vi "NI 9775 Continuous Mode 4 channels (Host).vi"() -> ()   [LabVIEW 2021]
uses:
  <vilib>/userDefined/High Color/nirio_resource_hc.ctl
  <vilib>/LabVIEW Targets/FPGA/cRIO/shared/nicrio_ModuleControls/nicrio_cRIO-9775_ContinuousDataRates4ChansRing.ctl
  <vilib>/LabVIEW Targets/FPGA/cRIO/shared/nicrio_ModuleControls/nicrio_BasicConversionTime.ctl
  <vilib>/FPGAPlugInAG/cRIO-9053/niLvFpga_Open_cRIO-9053.vi
  <vilib>/rvi/interface/common/dynamic/niFpgaDynamicAddResources.vi
  <vilib>/FPGAPlugInAG/Dynamic/niLvFpga_Reset_Dynamic.vi
  <vilib>/Utility/error.llb/Error Cluster From Error Code.vi
  <vilib>/rvi/errors/niLvFpgaAdjustHostInterfaceError.vi
  <vilib>/FPGAPlugInAG/Dynamic/niLvFpga_Run_Dynamic.vi
  <vilib>/Utility/file.llb/Write Delimited Spreadsheet (DBL).vi
  <vilib>/FPGAPlugInAG/Dynamic/niLvFpga_Close_Dynamic.vi
  <vilib>/rvi/interface/nirviOpenFPGA/nirviOpenFPGA.xnode
  FPGA Bitfiles/ni9775crio9053_FPGATarget2_NI9775GettingSta_I+1qGd-Sz4M.lvbitx
  <vilib>/rvi/interface/nirviMethod/nirviMethod.xnode
  <vilib>/rvi/interface/nirviReadWriteControl/nirviReadWriteControl.xnode
  <vilib>/rvi/interface/nirviCloseFPGA/nirviCloseFPGA.xnode
  <vilib>/rvi/interface/Simulation/niFpgaSimulationCallBeginRW.vi
  <vilib>/FPGAPlugInAG/Dynamic/niLvFpga_ReadFifo_Dynamic.vi
  <vilib>/rvi/errors/niLvFpgaMergeErrorWithErrorCode.vi
  NiFpgaLv.dll
panel:
  out "Num pts Pos":i32=50
  out "Modulation frequency":dbl=1000.0
  out "Sample Rate":dbl=100000.0
  out "Num pts Neg":i32=50
  out "Raw signal":waveform(dbl)[](graph)=[{"t0"=timestamp(0 s since 1904-01-01), "dt"=1e-05, "Y"=array[4941 elements]}, {"t0"=timestamp(0 s since 1904-01-01), "dt"=1e-05, "Y"=array[4941 elements]}, {"t0"=timestamp(0 s since 1904-01-01), "dt"=1e-05, "Y"=array[4941 elements]}, {"t0"=timestamp(0 s since 1904-01-01), "dt"=1e-05, "Y"=array[4941 elements]}]
  in  "Save modulated signal":bool=TRUE
  out "Producer loop time":u32=50
  out "Consumer loop time":u32=50
  in  "Filename":path=path "C:/Users/data/ni9775_100ks_1khz.lvm"
  in  "Consumer loop update rate (ms)":u32=10
  out "Demodulated Signal":dbl(graph)
  out "middle point pos":dbl=0.437255859375
  out "Queue":i32
  out "Original Signal middle":dbl(graph)=0.437255859375
  out "Low level":bool=TRUE
  out "High level":bool
  in  "Enable Low Pass Filter":T1={"Enable Low Pass Filter CH1"=TRUE, "Enable Low Pass Filter CH2"=TRUE, "Enable Low Pass Filter CH3"=TRUE, "Enable Low Pass Filter CH0"=TRUE}
  in  "Timing Mode":T2=enum."High Resolution"
  in  "Continuous Data Rate":T3=200 items=["1.000 MS/s (NI 9775)"=20, "833.333 KS/s (NI 9775)"=24, "714.286 KS/s (NI 9775)"=28, "625.000 KS/s (NI 9775)"=32, "555.556 KS/s (NI 9775)"=36, "500.000 KS/s (NI 9775)"=40, "454.545 KS/s (NI 9775)"=44, "416.667 KS/s (NI 9775)"=48, "384.615 KS/s (NI 9775)"=52, "357.143 KS/s (NI 9775)"=56, "333.333 KS/s (NI 9775)"=60, "312.500 KS/s (NI 9775)"=64, "294.118 KS/s (NI 9775)"=68, "277.778 KS/s (NI 9775)"=72, "263.158 KS/s (NI 9775)"=76, "250.000 KS/s (NI 9775)"=80, "238.095 KS/s (NI 9775)"=84, "227.273 KS/s (NI 9775)"=88, "217.391 KS/s (NI 9775)"=92, "208.333 KS/s (NI 9775)"=96, "200.000 KS/s (NI 9775)"=100, "192.308 KS/s (NI 9775)"=104, "185.185 KS/s (NI 9775)"=108, "178.571 KS/s (NI 9775)"=112, "172.414 KS/s (NI 9775)"=116, "166.667 KS/s (NI 9775)"=120, "161.290 KS/s (NI 9775)"=124, "156.250 KS/s (NI 9775)"=128, "151.515 KS/s (NI 9775)"=132, "147.059 KS/s (NI 9775)"=136, "142.857 KS/s (NI 9775)"=140, "138.889 KS/s (NI 9775)"=144, "135.135 KS/s (NI 9775)"=148, "131.579 KS/s (NI 9775)"=152, "128.205 KS/s (NI 9775)"=156, "125.000 KS/s (NI 9775)"=160, "121.951 KS/s (NI 9775)"=164, "119.048 KS/s (NI 9775)"=168, "116.279 KS/s (NI 9775)"=172, "113.636 KS/s (NI 9775)"=176, "111.111 KS/s (NI 9775)"=180, "108.696 KS/s (NI 9775)"=184, "106.383 KS/s (NI 9775)"=188, "104.167 KS/s (NI 9775)"=192, "102.041 KS/s (NI 9775)"=196, "100.000 KS/s (NI 9775)"=200, "50.000 KS/s (NI 9775)"=400, "33.333 KS/s (NI 9775)"=600, "25.000 KS/s (NI 9775)"=800, "20.000 KS/s (NI 9775)"=1000, "16.667 KS/s (NI 9775)"=1200, "14.286 KS/s (NI 9775)"=1400, "12.500 KS/s (NI 9775)"=1600, "11.111 KS/s (NI 9775)"=1800, "10.000 KS/s (NI 9775)"=2000, "9.091 KS/s (NI 9775)"=2200, "8.333 KS/s (NI 9775)"=2400, "7.692 KS/s (NI 9775)"=2600, "7.143 KS/s (NI 9775)"=2800, "6.667 KS/s (NI 9775)"=3000, "6.250 KS/s (NI 9775)"=3200, "5.882 KS/s (NI 9775)"=3400, "5.556 KS/s (NI 9775)"=3600, "5.000 KS/s (NI 9775)"=4000, "4.762 KS/s (NI 9775)"=4200, "4.545 KS/s (NI 9775)"=4400, "4.348 KS/s (NI 9775)"=4600, "4.167 KS/s (NI 9775)"=4800, "4.000 KS/s (NI 9775)"=5000, "3.846 KS/s (NI 9775)"=5200, "3.571 KS/s (NI 9775)"=5600, "3.333 KS/s (NI 9775)"=6000, "3.125 KS/s (NI 9775)"=6400, "2.941 KS/s (NI 9775)"=6800, "2.778 KS/s (NI 9775)"=7200, "2.632 KS/s (NI 9775)"=7600, "2.500 KS/s (NI 9775)"=8000, "2.381 KS/s (NI 9775)"=8400, "2.273 KS/s (NI 9775)"=8800, "2.174 KS/s (NI 9775)"=9200, "2.083 KS/s (NI 9775)"=9600, "2.000 KS/s (NI 9775)"=10000, "1.923 KS/s (NI 9775)"=10400, "1.852 KS/s (NI 9775)"=10800, "1.786 KS/s (NI 9775)"=11200, "1.724 KS/s (NI 9775)"=11600, "1.667 KS/s (NI 9775)"=12000, "1.613 KS/s (NI 9775)"=12400, "1.563 KS/s (NI 9775)"=12800, "1.515 KS/s (NI 9775)"=13200, "1.471 KS/s (NI 9775)"=13600, "1.429 KS/s (NI 9775)"=14000, "1.389 KS/s (NI 9775)"=14400, "1.351 KS/s (NI 9775)"=14800, "1.316 KS/s (NI 9775)"=15200, "1.282 KS/s (NI 9775)"=15600, "1.250 KS/s (NI 9775)"=16000, "1.220 KS/s (NI 9775)"=16400, "1.190 KS/s (NI 9775)"=16800, "1.163 KS/s (NI 9775)"=17200, "1.136 KS/s (NI 9775)"=17600, "1.111 KS/s (NI 9775)"=18000, "1.087 KS/s (NI 9775)"=18400, "1.064 KS/s (NI 9775)"=18800, "1.042 KS/s (NI 9775)"=19200, "1.020 KS/s (NI 9775)"=19600, "1.000 KS/s (NI 9775)"=20000, "0.980 KS/s (NI 9775)"=20400, "0.962 KS/s (NI 9775)"=20800, "0.943 KS/s (NI 9775)"=21200, "0.926 KS/s (NI 9775)"=21600, "0.909 KS/s (NI 9775)"=22000, "0.893 KS/s (NI 9775)"=22400, "0.877 KS/s (NI 9775)"=22800, "0.862 KS/s (NI 9775)"=23200, "0.847 KS/s (NI 9775)"=23600, "0.833 KS/s (NI 9775)"=24000, "0.820 KS/s (NI 9775)"=24400, "0.806 KS/s (NI 9775)"=24800, "0.794 KS/s (NI 9775)"=25200, "0.781 KS/s (NI 9775)"=25600, "0.694 KS/s (NI 9775)"=28800, "0.625 KS/s (NI 9775)"=32000, "0.568 KS/s (NI 9775)"=35200, "0.521 KS/s (NI 9775)"=38400, "0.446 KS/s (NI 9775)"=44800, "0.391 KS/s (NI 9775)"=51200, "0.347 KS/s (NI 9775)"=57600, "0.313 KS/s (NI 9775)"=64000]
  out "Host error out":errorcluster
  out "FPGA error out":errorcluster
  in  "stop":bool
  out "FIFO":u32=40
  out "Data FIFO Full":bool
  in  "Read FIFO update rate (ms)":u32=50
  in  "RIO Device":T4="RIO0"
  # "Overview: Acquire signals from NI 9775 and demodulate the photodiode.\nRequirements: LabVIEW Full Development System, LV FPGA, and NI RIO\nInstructions: \n1. Run the VI."
  # "FPGA Input Parameters"
  # "Timing Parameters"
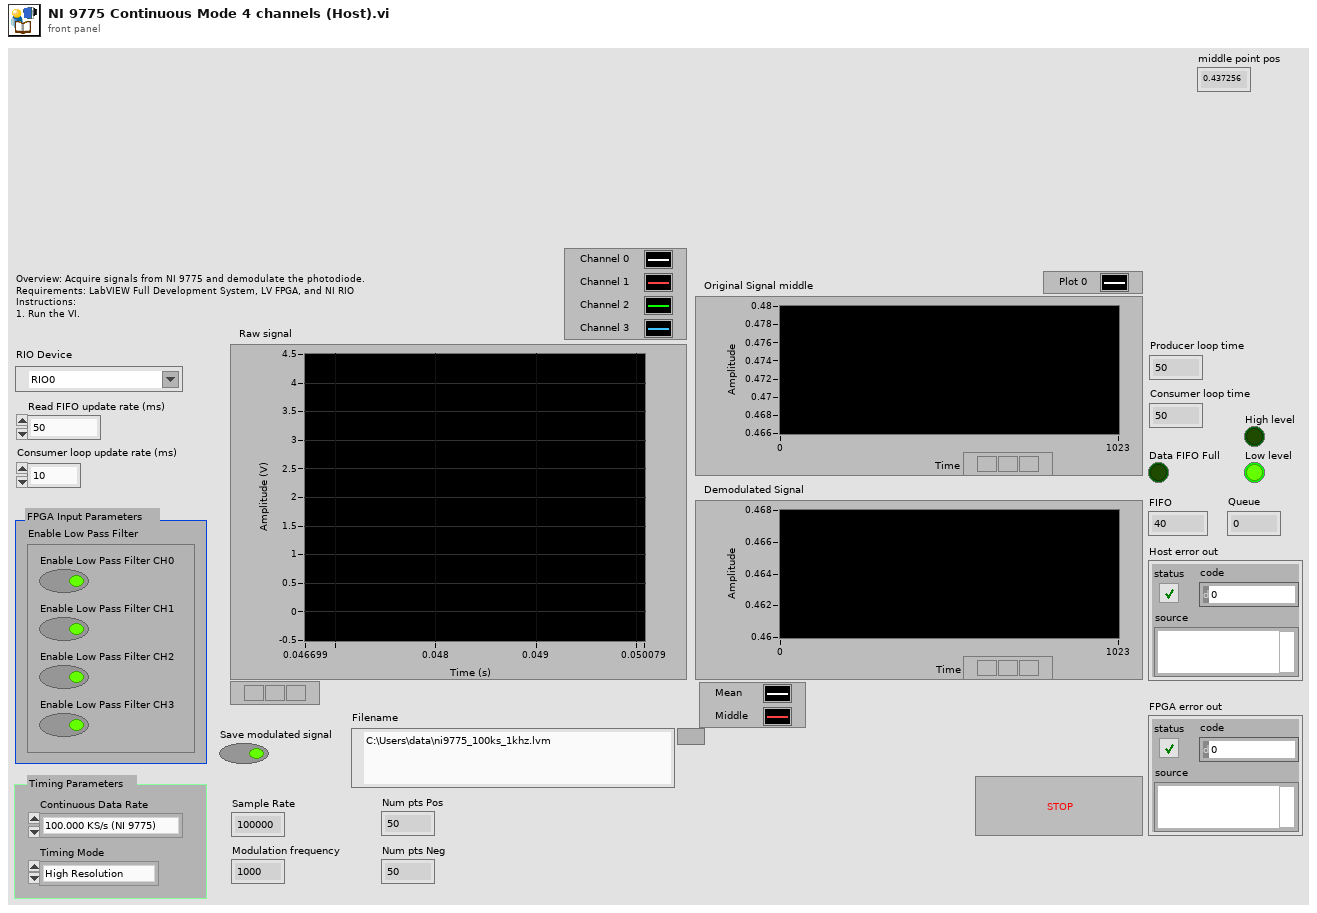
[diagram p1: front panel]
types:
  T1 = cluster{"Enable Low Pass Filter CH1":bool, "Enable Low Pass Filter CH2":bool, "Enable Low Pass Filter CH3":bool, "Enable Low Pass Filter CH0":bool}
  T2 = typedef "nicrio_BasicConversionTime.ctl" = enum8{"High Speed", "High Resolution"}
  T3 = typedef "nicrio_cRIO-9775_ContinuousDataRates4ChansRing.ctl" = u16
  T4 = typedef "nirio_resource_hc.ctl" = tag
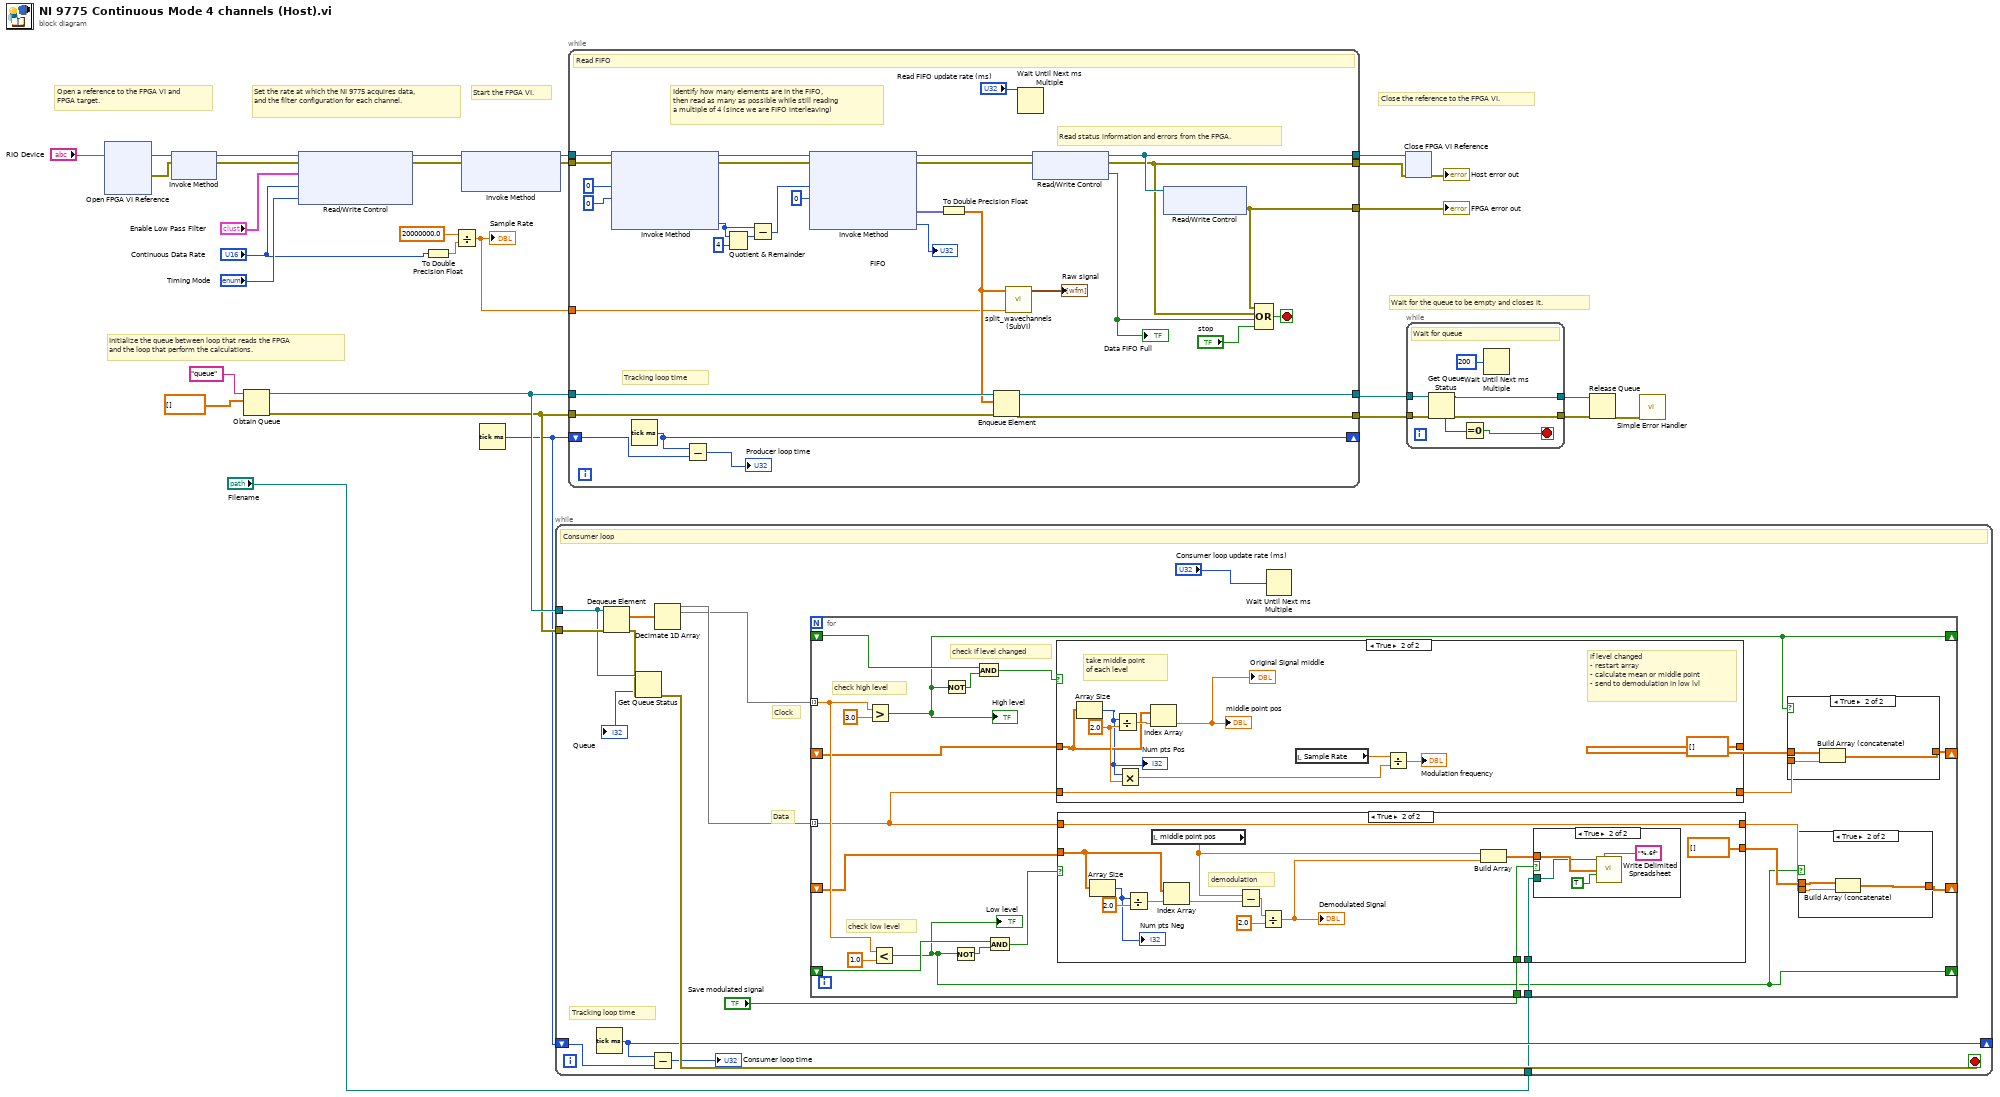
[diagram p0: block diagram]
diagram:
  # "Initialize the queue between loop that reads the FPGA\nand the loop that perform the calculations."
  # "Wait for the queue to be empty and closes it."
  # "Close the reference to the FPGA VI."
  # "Start the FPGA VI."
  # "Set the rate at which the NI 9775 acquires data, and the filter configuration for each channel."
  # "Open a reference to the FPGA VI and FPGA target."
  n1 = xnode "Open FPGA VI Reference"("resource name"="RIO Device") -> ("FPGA VI Reference Out"=w18:refnum<k20>, "error out"=w17:errorcluster)  [unwired: 1 in]
  n2 = xnode "Invoke Method"("FPGA VI Reference In"=w18, "error in"=w17) -> ("FPGA VI Reference Out"=w22:refnum<k20>, "error out"=w23:errorcluster)
  n3 = Obtain Queue(name (unnamed)="queue", element data type=dbl[] []) -> (queue out=w13:refnum<queue>, error out=w10:errorcluster)  [unwired: 3 in, 1 out]
  n4 = xnode "Read/Write Control"("FPGA VI Reference In"=w22, "error in"=w23, "Enable Low Pass Filter"="Enable Low Pass Filter", "Continuous Data Rate"="Continuous Data Rate", "Timing Mode"="Timing Mode") -> ("FPGA VI Reference Out"=w26:refnum<k20>, "error out"=w27:errorcluster)
  n5 = To Double Precision Float(number="Continuous Data Rate") -> (double precision float=w3:dbl)
  n6 = Divide(x=20000000.0, y=w3) -> (x/y=w1:dbl)
  "Sample Rate" <- w1
  n7 = xnode "Invoke Method"("FPGA VI Reference In"=w26, "error in"=w27) -> ("FPGA VI Reference Out"=w29:refnum<k20>, "error out"=w30:errorcluster)  [unwired: 1 in]
  n8 = Tick Count (ms)() -> (millisecond timer value=w6:u32)
  n9 = while {
    tunnel: w13 -> [w42]
    tunnel: w10 -> [w44]
    shift-right: [w36] -> _
    shift-left: w6 -> [w35]
    tunnel: "Filename" -> [w32]
    stop <- w40 stop-if-true
    # "Tracking loop time"
    # "Data"
    # "Clock"
    # "Consumer loop"
    n10 = Tick Count (ms)() -> (millisecond timer value=w36:u32)
    n11 = Dequeue Element(queue=w42, error in (no error)=w44) -> (element=w31:dbl[], error out=w41:errorcluster)  [unwired: 1 in, 2 out]
    n12 = Get Queue Status(queue=w42, error in (no error)=w41) -> (error out=w40:errorcluster, # elements in queue=→"Queue":i32)  [unwired: 1 in, 6 out]
    n13 = Subtract(x=w36, y=w35) -> (x-y=→"Consumer loop time":u32)
    n14 = Decimate 1D Array(w31) -> (w43:dbl[], w38:dbl[])  [unwired: 2 out]
    n15 = for {
      tunnel: w38 -> [w61] mode=indexing
      shift-right: [w46] -> _
      shift-left: _ -> [w60]
      shift-right: [w45] -> _
      shift-left: _ -> [w62]
      shift-right: [w56] -> _
      shift-left: _ -> [w59]
      shift-right: [w57] -> _
      shift-left: _ -> [w58]
      tunnel: w43 -> [w51] mode=indexing
      tunnel: "Save modulated signal" -> [w50]
      tunnel: w32 -> [w49]
      # "check low level"
      # "check high level"
      # "check if level changed"
      n16 = Greater?(x=w61, y=3.0) -> (0:w46:bool)
      "High level" <- w46
      n17 = Less?(x=w61, y=1.0) -> (x < y?=w45:bool)
      "Low level" <- w45
      n18 = Not(x=w46) -> (.not. x?=w65:bool)
      n19 = Not(x=w45) -> (.not. x?=w63:bool)
      n20 = And(x=w60, y=w65) -> (x .and. y?=w48:bool)
      n21 = And(x=w62, y=w63) -> (x .and. y?=w47:bool)
      n22 = case shown="True" w48 {
        tunnel: [w68 dbl[] []] -> w54
        tunnel: w58 -> [w68 w71]
        tunnel: [w67 w78] -> w53
        tunnel: w51 -> [w67 w78]
        frame False {
        }
        frame True {
          w76 = 2.0 ("y")
          # "if level changed\n- restart array\n- calculate mean or middle point\n- send to demodulation in low lvl"
          # "take middle point \nof each level"
          n23 = Array Size(array=w71) -> (size(s)=w70:i32)
          "Num pts Pos" <- w70
          n24 = Divide(x=w70, y=w76) -> (x/y=w72:dbl)
          n25 = Multiply(x=w70, y=w76) -> (x*y=w74:dbl)
          n26 = Index Array(array=w71, index=w72) -> (element=→"Original Signal middle" →"middle point pos":dbl)
          n27 = local read "Sample Rate"() -> (w75:dbl)
          n28 = Divide(x=w75, y=w74) -> (x/y=→"Modulation frequency":dbl)
        }
      }
      n29 = case shown="True" w47 {
        tunnel: [w80 dbl[] []] -> w55
        tunnel: w59 -> [w80 w83]
        tunnel: [w79 w94] -> w52
        tunnel: w51 -> [w79 w94]
        tunnel: w50 -> [_ w88]
        tunnel: w49 -> [_ w86]
        frame False {
        }
        frame True {
          # "demodulation"
          n30 = Array Size(array=w83) -> (size(s)=w85:i32)
          "Num pts Neg" <- w85
          n31 = Divide(x=w85, y=2.0) -> (x/y=w84:dbl)
          n32 = local read "middle point pos"() -> (w81:dbl)
          n33 = Index Array(array=w83, index=w84) -> (element=w90:dbl)
          n34 = Subtract(x=w81, y=w90) -> (x-y=w92:dbl)
          n35 = Divide(x=w92, y=2.0) -> (x/y=w82:dbl)
          "Demodulated Signal" <- w82
          n36 = Build Array(w81, w82) -> (w87:dbl[])
          n37 = case shown="True" w88 {
            tunnel: w87 -> [_ w97]
            tunnel: w86 -> [_ w96]
            frame False {
            }
            frame True {
              n38 = call-poly <vilib>:"Write Delimited Spreadsheet.vi"("file path (dialog if empty)"=w96, "format (%.3f)"="%.6f", "1D data"=w97, "append to file? (new file:F)"=TRUE) -> ()  [unwired: 10 in, 2 out]
            }
          }
        }
      }
      n39 = case shown="True" w46 {
        tunnel: w54 -> [w103 w106]
        tunnel: [w103 w104] -> w57
        tunnel: w53 -> [_ w105]
        frame False {
        }
        frame True {
          n40 = Build Array (concatenate)(w106, w105) -> (w104:dbl[])
        }
      }
      n41 = case shown="True" w45 {
        tunnel: w55 -> [w99 w102]
        tunnel: w52 -> [_ w101]
        tunnel: [w99 w100] -> w56
        frame False {
        }
        frame True {
          n42 = Build Array (concatenate)(w102, w101) -> (w100:dbl[])
        }
      }
    }
    n43 = Wait Until Next ms Multiple(millisecond multiple="Consumer loop update rate (ms)") -> ()  [unwired: 1 out]
  }
  n44 = while {
    tunnel: w30 -> [w121]
    tunnel: w29 -> [w122]
    tunnel: [w130] -> w28
    tunnel: [w129] -> w25
    tunnel: [w128] -> w21
    tunnel: w13 -> [w116]
    tunnel: [w115] -> w12
    tunnel: w10 -> [w114]
    tunnel: [w113] -> w9
    shift-right: [w111] -> _
    shift-left: w6 -> [w110]
    tunnel: w1 -> [w107]
    stop <- w138 stop-if-true
    # "Tracking loop time"
    # "Read status information and errors from the FPGA."
    # "Identify how many elements are in the FIFO, \nthen read as many as possible while still reading\na multiple of 4 (since we are FIFO interleaving)"
    # "Read FIFO"
    n45 = xnode "Invoke Method"("FPGA VI Reference In"=w122, "error in"=w121, "Number of Elements"=u32 0, "Timeout (ms)"=0) -> ("FPGA VI Reference Out"=w120:refnum<k20>, "error out"=w119:errorcluster, "Elements Remaining"=w123:u32)  [unwired: 1 out]
    n46 = Tick Count (ms)() -> (millisecond timer value=w111:u32)
    n47 = Subtract(x=w111, y=w110) -> (x-y=→"Producer loop time":u32)
    n48 = Quotient & Remainder(x=w123, y=u32 4) -> (x-y*floor(x/y)=w124:u32)  [unwired: 1 out]
    n49 = Subtract(x=w123, y=w124) -> (x-y=w118:u32)
    n50 = xnode "Invoke Method"("FPGA VI Reference In"=w120, "error in"=w119, "Number of Elements"=w118, "Timeout (ms)"=0 ("Timeout")) -> ("FPGA VI Reference Out"=w135:refnum<k20>, "error out"=w134:errorcluster, "Data"=w131:fxp<+/-,17,5>[], "Elements Remaining"=→"FIFO":u32)
    n51 = To Double Precision Float(number=w131) -> (double precision float=w108:dbl[])
    n52 = Enqueue Element(queue=w116, element=w108, error in (no error)=w114) -> (queue out=w115:refnum<queue>, error out=w113:errorcluster)  [unwired: 1 in, 1 out]
    n53 = call "split_wavechannels (SubVI).vi"("Sample rate"=w107, "Array in"=w108) -> ("Array out"=→"Raw signal":waveform(dbl)[])  [unwired: 9 in]
    n54 = Wait Until Next ms Multiple(millisecond multiple="Read FIFO update rate (ms)") -> ()  [unwired: 1 out]
    n55 = xnode "Read/Write Control"("FPGA VI Reference In"=w135, "error in"=w134) -> ("FPGA VI Reference Out"=w130:refnum<k20>, "error out"=w129:errorcluster, "Data FIFO Full"=w137:bool)
    "Data FIFO Full" <- w137
    n56 = xnode "Read/Write Control"("FPGA VI Reference In"=w130) -> ("FPGA Error Out"=w128:errorcluster)  [unwired: 1 in, 2 out]
    n57 = Compound Arithmetic op=OR(w128, w129, w137, "stop") -> (w138:bool)
  }
  "FPGA error out" <- w21
  n58 = xnode "Close FPGA VI Reference"("FPGA VI Reference In"=w28, "error in"=w25) -> ("error out"=→"Host error out":errorcluster)
  n59 = while {
    tunnel: w12 -> [w145]
    tunnel: [w141] -> w11
    tunnel: w9 -> [w140]
    tunnel: [w139] -> w8
    stop <- w143 stop-if-true
    # "Wait for queue"
    n60 = Get Queue Status(queue=w145, error in (no error)=w140) -> (queue out=w141:refnum<queue>, error out=w139:errorcluster, # elements in queue=w144:i32)  [unwired: 1 in, 5 out]
    n61 = Equal To 0?(x=w144) -> (x = 0?=w143:bool)
    n62 = Wait Until Next ms Multiple(millisecond multiple=u32 200) -> ()  [unwired: 1 out]
  }
  n63 = Release Queue(queue=w11, error in (no error)=w8) -> (error out=w7:errorcluster)  [unwired: 1 in, 2 out]
  n64 = call <vilib>:"Simple Error Handler.vi"("error in (no error)"=w7) -> ()  [unwired: 4 in, 5 out]
